vi "KV_CurHead_Addr_Reset.vi"() -> (3 "OK?":bool)   [LabVIEW 2015]
uses:
  <vilib>/Instr/_visa.llb/VISA Configure Serial Port (Instr).vi
panel:
  in  "MyIndex":u8
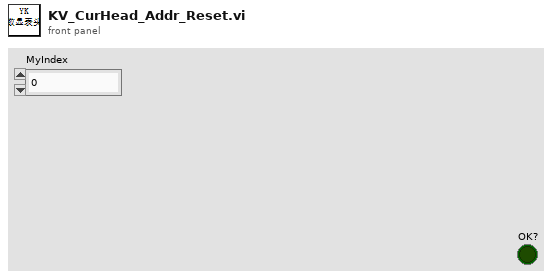
[diagram p1: front panel]
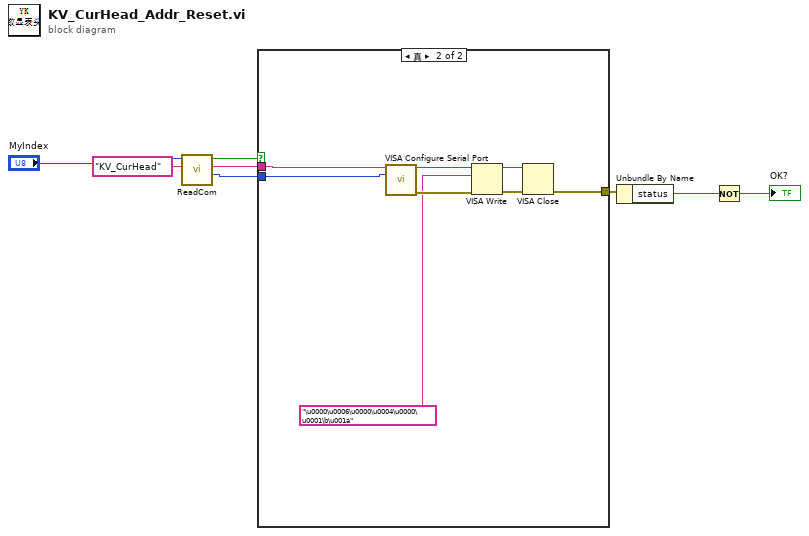
[diagram p0: block diagram]
diagram:
  n1 = call "ReadCom.vi"("仪器名称"="KV_CurHead", "MyIndex"="MyIndex") -> ("Baudrate"=w1:i32, "COM"=w2:string, "OK?"=w3:bool)  [unwired: 7 in]
  n2 = case shown="真" w3 {
    tunnel: [_ w11] -> w8
    tunnel: w2 -> [_ w12]
    tunnel: w1 -> [_ w9]
    frame False {
    }
    frame True {
      n3 = call-poly "VISA Configure Serial Port"("VISA resource name"=w12, "baud rate (9600)"=w9) -> ("VISA resource name out"=w16:refnum<visa-resource-name>, "error out"=w15:errorcluster)  [unwired: 12 in]
      n4 = VISA Write(VISA resource name=w16, write buffer="\u0000\u0006\u0000\u0004\u0000\u0001\b\u001a", error in (no error)=w15) -> (VISA resource name out=w10:refnum<visa-resource-name>, error out=w13:errorcluster)  [unwired: 1 out]
      n5 = VISA Close(VISA resource name=w10, error in (no error)=w13) -> (error out=w11:errorcluster)
    }
  }
  n6 = Unbundle By Name(w8) -> ("status"=w7:bool)
  n7 = Not(x=w7) -> (.not. x?=→"OK?":bool)
